vi "Get All VI refnums.vi"(8 "error in (no error)":errorcluster, 11 "DebuggingTerminal in":refnum<class "DebuggingTerminal.lvclass">) -> (0 "error out":errorcluster, 2 "refnums":refnum<vi>[](array[refnum]), 3 "DebuggingTerminal out":refnum<class "DebuggingTerminal.lvclass">)   [LabVIEW 2013, in "MQTT Base.lvlib" / "DebuggingTerminal.lvclass"]
uses:
  DebuggingTerminal.lvclass
  DebuggingTerminal.lvclass/DebuggingTerminal.ctl
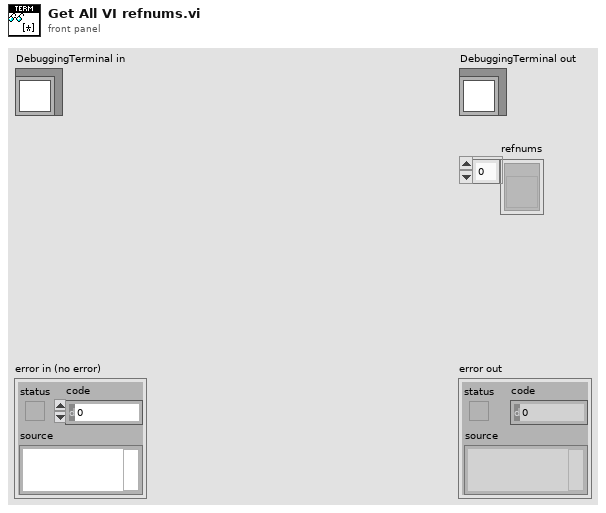
[diagram p1: front panel]
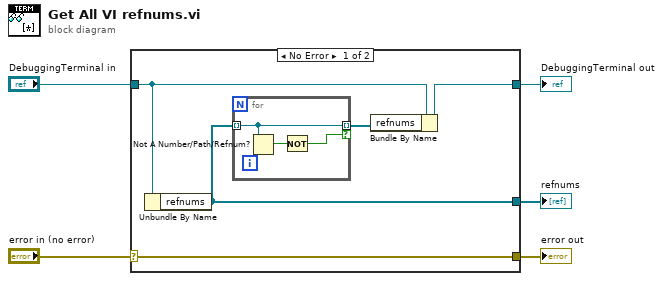
[diagram p0: block diagram]
diagram:
  n1 = case shown="No Error" "error in (no error)" {
    selector: "error in (no error)" -> [w10 w14]
    tunnel: [w10 w14] -> w4
    tunnel: [w6 w15] -> w2
    tunnel: "DebuggingTerminal in" -> [w7 w15]
    tunnel: [w9 _] -> w1
    frame No Error {
      n2 = Unbundle By Name(w7) -> ("refnums"=w9:refnum<vi>[])
      n3 = for {
        tunnel: w9 -> [w13] mode=indexing
        tunnel: [w13] -> w8 mode=indexing if=w11
        n4 = Not A Number/Path/Refnum?(number/path/refnum=w13) -> (NaN/Path/Refnum?=w12:bool)
        n5 = Not(x=w12) -> (.not. x?=w11:bool)
      }
      n6 = Bundle By Name(cluster=w7, "refnums"=w8) -> (w6:refnum<class "DebuggingTerminal.lvclass">)
    }
    frame Error {
    }
  }
  "error out" <- w4
  "DebuggingTerminal out" <- w2
  "refnums" <- w1
